vi "DUAL GAUGE-RW Toor lock.vi"(7 "W/R":bool, 8 "Fehler (Eingang)":errorcluster, 9 "Set Toor lock":i32(ring) items=["off (default)", " on"], 11 "Referenz in":refnum<visa-resource-name>) -> (0 "Cluster (Ausgang)":errorcluster, 1 "Get Toor lock":i32(ring) items=["off (default)", " on"], 3 "Referenz out":refnum<visa-resource-name>)   [LabVIEW 2010, in "Dual Gauge.lvlib"]
uses:
  Dual Gauge.lvlib
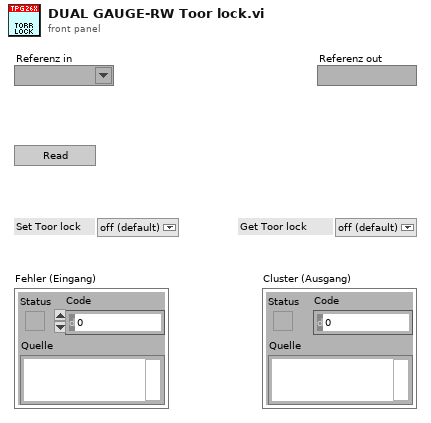
[diagram p1: front panel]
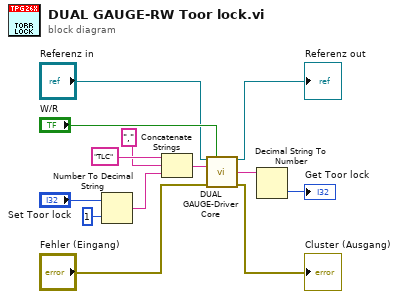
[diagram p0: block diagram]
diagram:
  n1 = Number To Decimal String(number="Set Toor lock", width (-)=i16 1) -> (decimal integer string=w9:string)
  n2 = Concatenate Strings("TLC" ("Command"), "," ("Command"), w9) -> (w5:string)
  n3 = call "DUAL GAUGE-Driver Core.vi"("Referenz in"="Referenz in", "Write/Read"="W/R", "Command"=w5, "Fehler (Eingang)"="Fehler (Eingang)") -> ("Referenz out"=→"Referenz out":refnum<visa-resource-name>, "String Out"=w7:string, "Cluster (Ausgang)"=→"Cluster (Ausgang)":errorcluster)  [unwired: 9 in]
  n4 = Decimal String To Number(string=w7) -> (number=→"Get Toor lock":i32)  [unwired: 2 in, 1 out]
